vi "pxie_7962_dram_as_memory_fpga.vi"() -> ()   [LabVIEW 2014]
uses:
  <vilib>/Platform/TimedLoop/XDataNode/XDataNode.xnode
  <vilib>/Platform/TimedLoop/XDataNode/nitl_modes.ctl
  <vilib>/Platform/TimedLoop/XDataNode/XDNodeRunTimeDep.lvlib
  <vilib>/Platform/TimedLoop/XDataNode/wakeup.ctl
  <vilib>/Platform/TimedLoop/XDataNode/timing_clust.ctl
  <instrlib>/_niInstr/Streaming/v1/FPGA/niInstr Streaming v1 FPGA.lvlib
  <vilib>/rvi/DataTransferAndStorage/Container/XNode/niFpgaContainer.xnode
  <vilib>/rvi/FIFO/Fifo_Resource/niFpgaFifoEmulationRefIn.vi
  FPGA_Controls/Acquisition FIFOs Cluster.ctl
  <vilib>/eio/EIONode/EIONode.xnode
  <vilib>/rvi/eio/common/nirviEmuTemplateMethod_errors.vi
  <instrlib>/_niInstr/Basic Elements/v1/FPGA/niInstr Basic Elements v1 FPGA.lvlib
  <instrlib>/_niInstr/Streaming/v1/Common/Stream State.ctl
  <instrlib>/_niInstr/Streaming/v1/Common/niInstr Streaming v1 Common.lvlib
  <instrlib>/_niInstr/Basic Elements/v1/FPGA/Private/Count Up U64.vi
  <vilib>/rvi/interface/RandomDataEmulation/nirviRandomDataFpgaReadWriteTemplate.vi
  <vilib>/rvi/FIFO/Fifo_Resource/nirvififoEmulationWrite.vi
panel:
  in  "trigger \ncount":u64
  in  "Clear Trigger":bool
  in  "Debug":bool
  out "stream.metadata 0":u64
  in  "stream.request state 0":T1
  out "stream.samples transferred 0":u64
  out "stream.state 0":T1
  in  "stream.num samples 0":u64
  out "stream 1 \nidle state":bool
  out "stream 1 finite\ntransfer state":bool
  out "stream 1\ncancel state":bool
  out "stream 1\nnot ready state":bool
  out "stream 1\nerror state":bool
  out "Stream 1 data invalid":bool
  out "Writes to DMA":u64
  out "Writes to bundeling FIFO":u64
  out "Samples Aquired":u64
  out "Init Done":bool
  in  "stream.num samples 1":u64
  out "stream.state 1":T1
  out "stream.samples transferred 1":u64
  in  "stream.request state 1":T1
  out "stream.metadata 1":u64
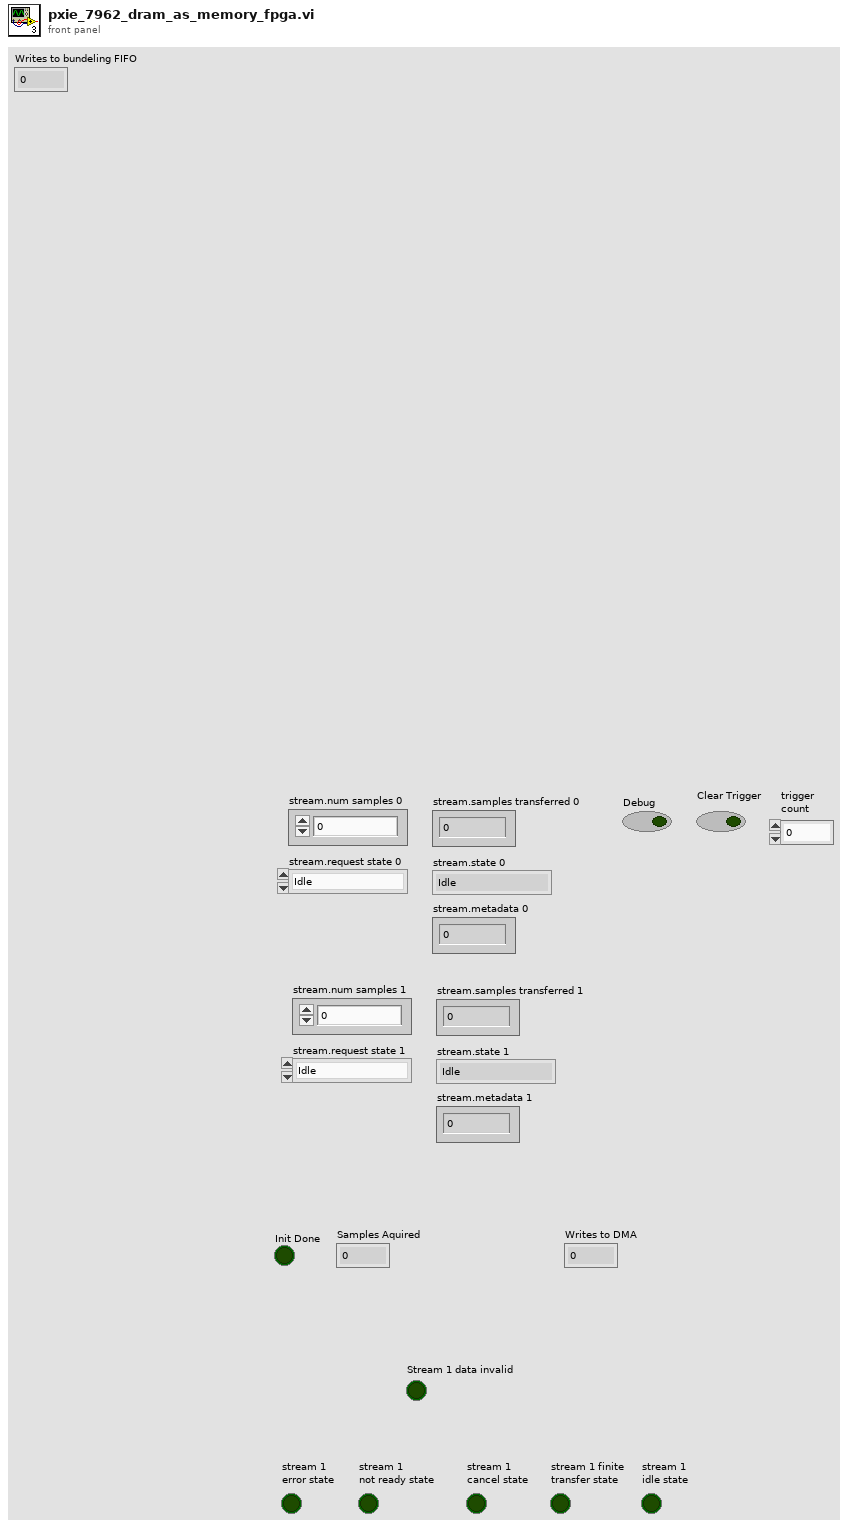
[diagram p1: front panel]
types:
  T1 = typedef "niInstr Streaming v1 Common.lvlib/Stream State.ctl" = enum8{"Idle", "Finite Transfer", "Continuous", "Done", "Error", "Not Ready", "Cancel"}
  T2 = typedef "XDNodeRunTimeDep.lvlib/timing_clust.ctl" = cluster{"Expected End [f-1]":u64, "Actual End [f-1]":u64, "Finished Late? [f-1]":bool, "Expected End [i-1]":u64, "Actual End [i-1]":u64, "Finished Late? [i-1]":bool, "Expected Start [i]":u64, "Actual Start [i]":u64, "Expected Start [f]":u64, "Actual Start [f]":u64, "Source Name":string, "Structure Name":string, "Period":i64, "Deadline":i64, "Offset":i64, "Start":i64, "Priority":i32, "Timeout":i32, "Mode":T3, "Wakeup Reason":T4, "Error":errorcluster, "Source Type":string, "Secondary Source Type":string, "Global End Time":u64, "Global Start Time":u64, "Frame Duration":u64, "Iteration Duration":u64, "Assigned CPU":i32, "I/O Scan Engine Mode":u32}
  T3 = typedef "XDNodeRunTimeDep.lvlib/nitl_modes.ctl" = enum32{"No Change", "Process missed periods, maintain original phase", "Discard missed periods, maintain original phase", "Process missed periods, ignore original phase", "Discard missed periods, ignore original phase"}
  T4 = typedef "XDNodeRunTimeDep.lvlib/wakeup.ctl" = enum32{"Normal", "Aborted", "Asynchronous wakeup", "Timing source error", "Timed loop error", "Timeout"}
  T5 = typedef "Acquisition FIFOs Cluster.ctl" = cluster{"FIFO 0":refnum<k21>, "FIFO 1":refnum<k21>, "FIFO 2":refnum<k21>, "FIFO 3":refnum<k21>, "FIFO 4":refnum<k21>, "FIFO 5":refnum<k21>, "FIFO 6":refnum<k21>, "FIFO 7":refnum<k21>}
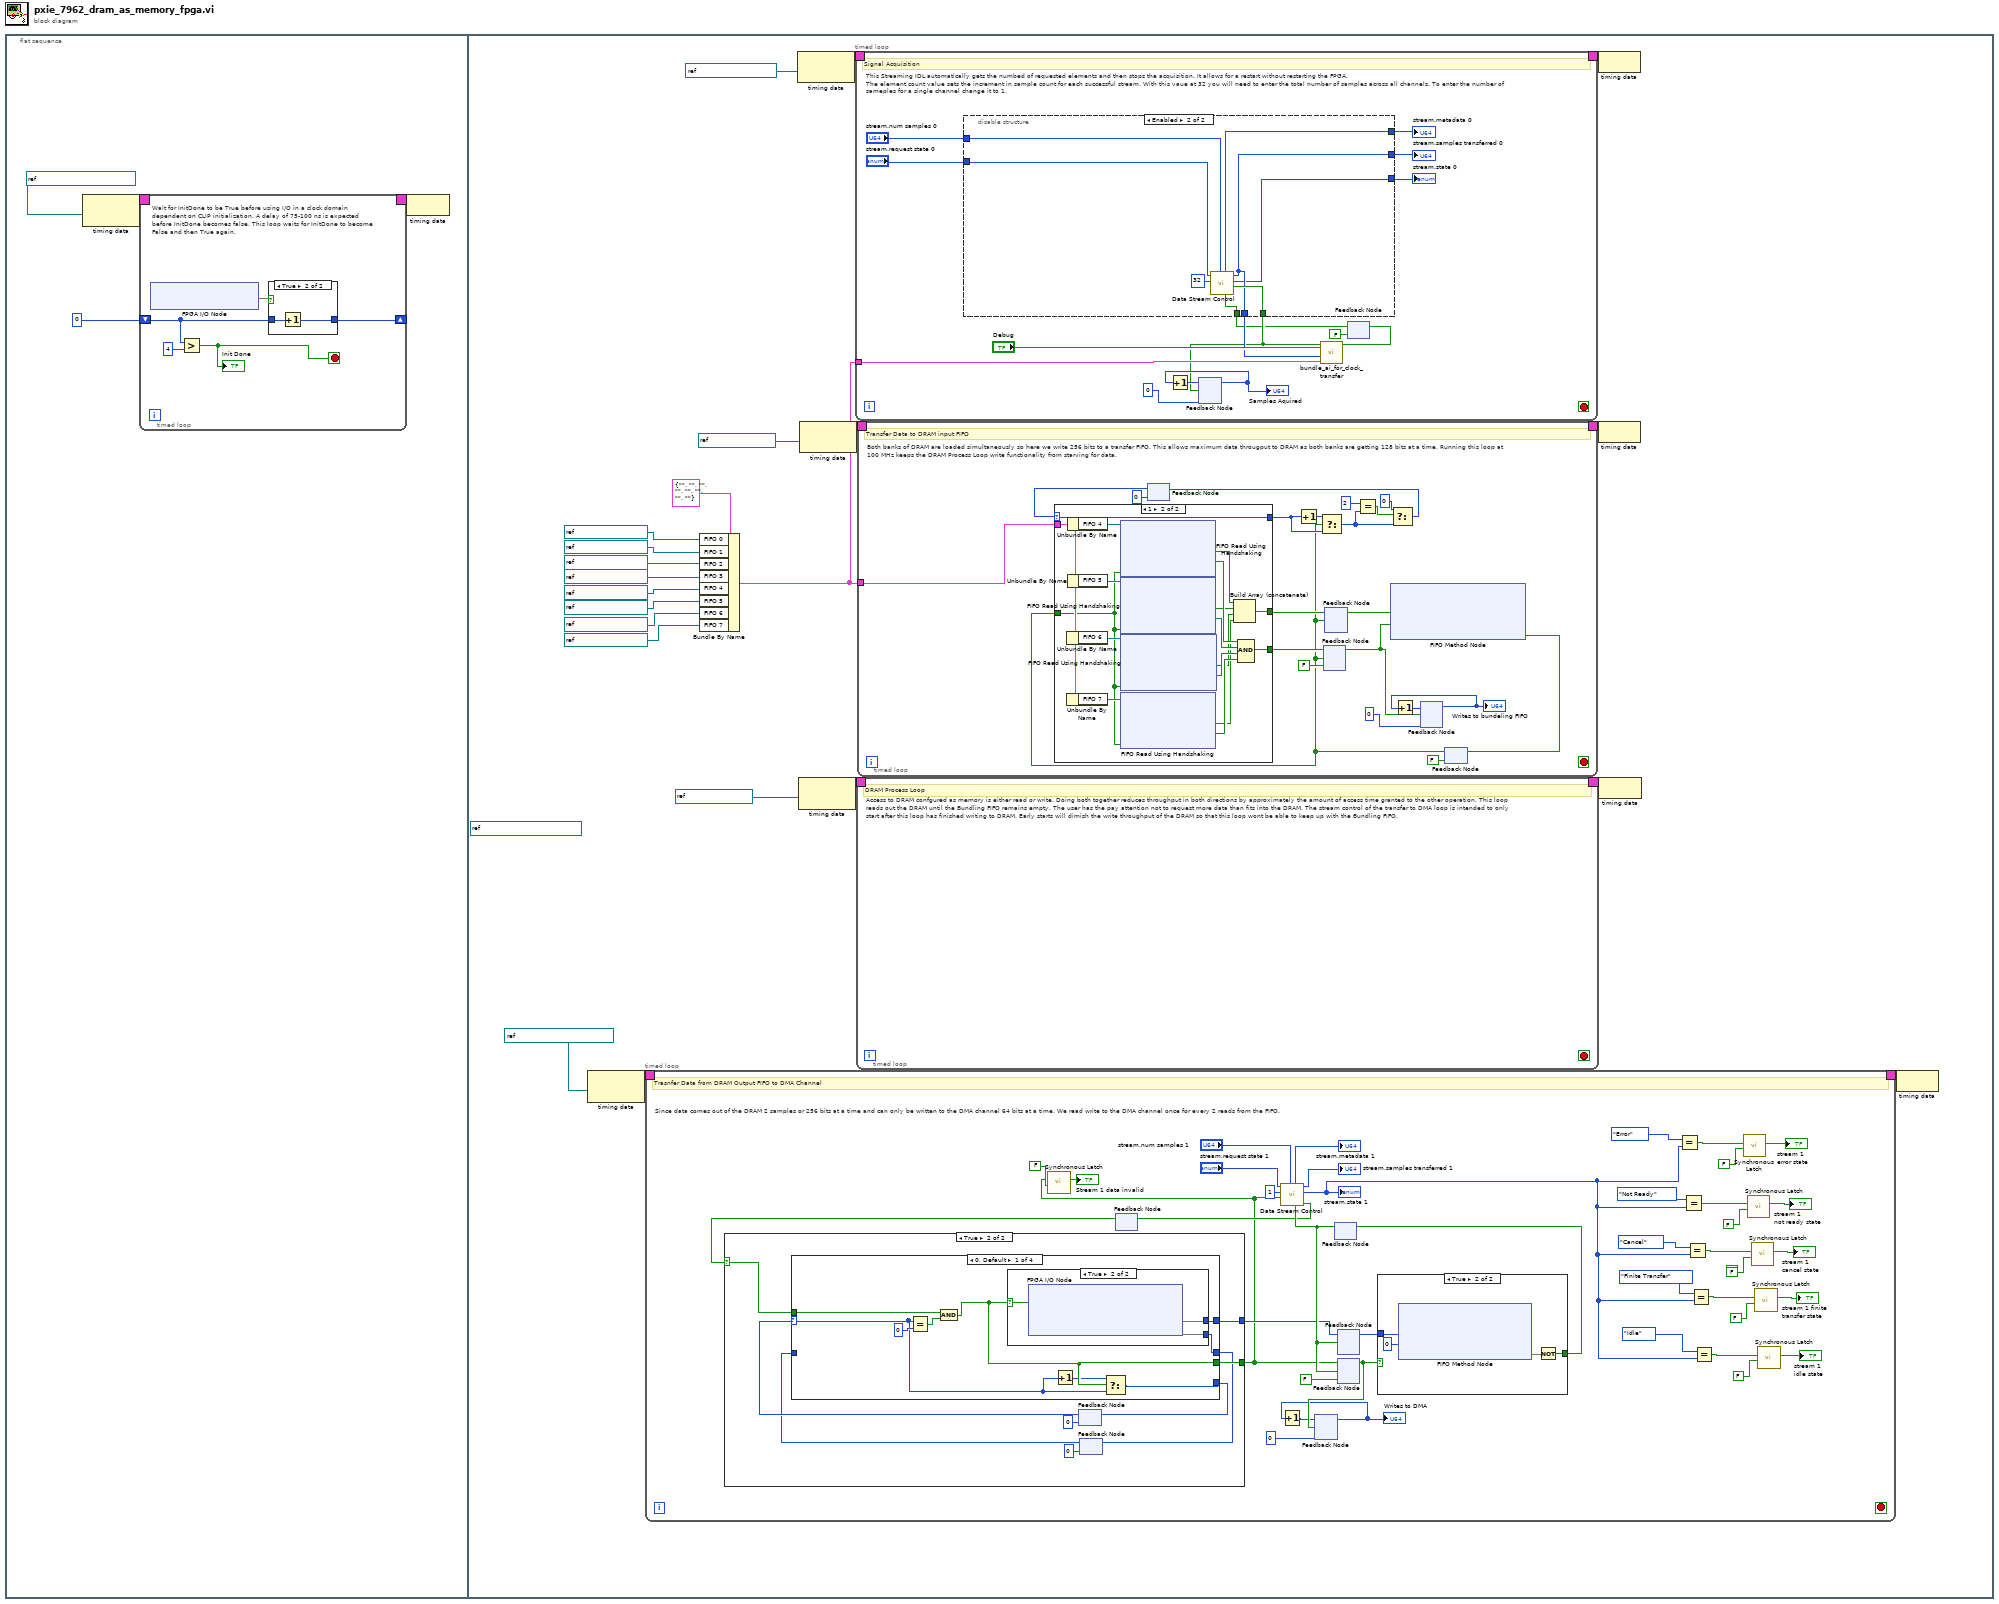
[diagram p0: block diagram]
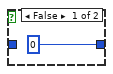
[diagram p2: hidden frame]
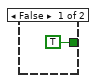
[diagram p3: hidden frame]
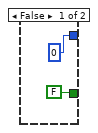
[diagram p4: hidden frame]
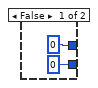
[diagram p5: hidden frame]
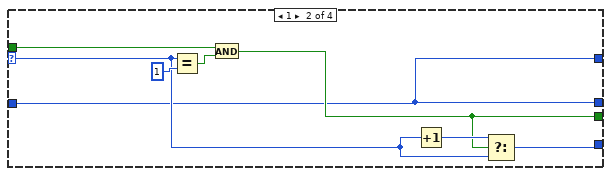
[diagram p6: hidden frame]
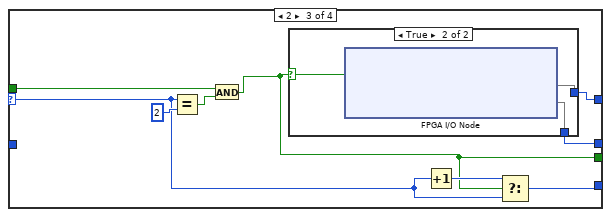
[diagram p7: hidden frame]
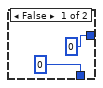
[diagram p8: hidden frame]
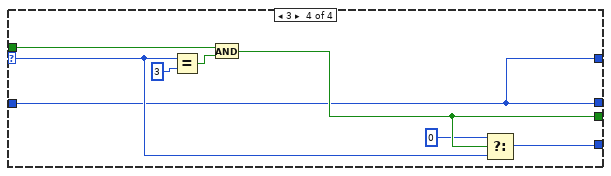
[diagram p9: hidden frame]
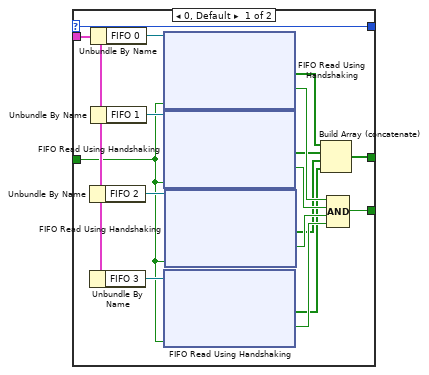
[diagram p10: hidden frame]
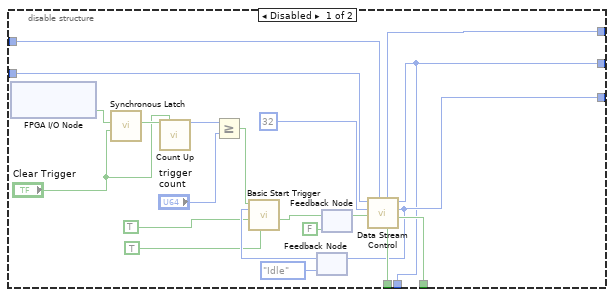
[diagram p11: hidden frame]
diagram:
  n1 = flat-sequence {
    frame #0 {
      n2 = node-c288(refnum<k21> "40 MHz Onboard Clock" ("Source Name")) -> (w4:T2)
      n3 = timed-loop {
        shift-right: [w8] -> _
        shift-left: u16 0 -> [w7]
        timing: w4 -> [_]
        timing-out: [_] -> w3
        stop <- w5 stop-if-true
        # "Wait for InitDone to be True before using I/O in a clock domain dependent on CLIP initialization. A delay of 75-100 ns is expected before InitDone becomes false. This loop waits for InitDone to become False and then True again."
        n4 = xnode "FPGA I/O Node"() -> ("IO Module\\InitDone"=w9)  [unwired: 1 in, 1 out]
        n5 = Greater?(x=w7, y=u16 4) -> (0:w5:bool)
        "Init Done" <- w5
        n6 = case shown="True" w9 {
          tunnel: [u16 0 w12] -> w8
          tunnel: w7 -> [_ w11]
          frame False {
          }
          frame True {
            n7 = Increment(x=w11) -> (x+1=w12:u16)
          }
        }
      }
      n8 = node-c288(w3) -> ()
    }
    frame #1 {
      (unwired) refnum<k21> "Bundling to DRAM FIFO" ("FIFO In")
      n9 = node-c288(refnum<k21> "40 MHz Onboard Clock" ("Source Name")) -> (w34:T2)
      n10 = timed-loop {
        timing: w34 -> [_]
        timing-out: [_] -> w33
        stop <- _ stop-if-true
        (unwired) FALSE ("clear")
        # "Since data comes out of the DRAM 2 samples or 256 bits at a time and can only be written to the DMA channel 64 bits at a time. We read write to the DMA channel once for every 2 reads from the FIFO."
        # "Trasnfer Data from DRAM Output FIFO to DMA Channel"
        n11 = feedback #1() -> (w71:bool)  [unwired: 1 in]
        n12 = case shown="True" w71 {
          selector: w71 -> [_ w92]
          tunnel: [u64 0 ("DRAM Bank 1\\Read_Data_Lower") w96] -> w69
          tunnel: [FALSE w91] -> w62
          frame False {
          }
          frame True {
            n13 = feedback #2(i16 0) -> (w94:i16)
            n14 = feedback #3(u64 0 ("DRAM Bank 1\\Read_Data_Lower")) -> (w89:u64)
            n15 = case shown="0, Default" w94 {
              selector: w94 -> [w98 w113 w120 w135]
              tunnel: w92 -> [w103 w116 w125 w138]
              tunnel: [w102 w111 w124 w133] -> w96
              tunnel: [w101 w112 w122 w134] -> w95
              tunnel: [w100 w114 w121 w137] -> w91
              tunnel: [w97 w111 w119 w133] -> w90
              tunnel: w89 -> [_ w111 _ w133]
              frame 0, Default {
                n16 = Equal?(x=w98, y=i16 0) -> (x = y?=w104:bool)
                n17 = And(x=w103, y=w104) -> (x .and. y?=w100:bool)
                n18 = case shown="True" w100 {
                  selector: w100 -> [_ w109]
                  tunnel: [u64 0 ("DRAM Bank 0\\Read_Data_Upper") w110] -> w102
                  tunnel: [u64 0 ("DRAM Bank 0\\Read_Data_Lower") w108] -> w97
                  frame False {
                  }
                  frame True {
                    n19 = xnode "FPGA I/O Node"("DRAM Bank 0\\Read"=w109) -> ("DRAM Bank 0\\Read_Data_Upper"=w110, "DRAM Bank 0\\Read_Data_Lower"=w108)  [unwired: 3 in, 3 out]
                  }
                }
                n20 = Increment(x=w98) -> (x+1=w99:i16)
                n21 = Select(t=w99, s=w100, f=w98) -> (s? t:f=w101:i16)
              }
              frame 1 {
                n22 = Equal?(x=w113, y=i16 1) -> (x = y?=w117:bool)
                n23 = And(x=w116, y=w117) -> (x .and. y?=w114:bool)
                n24 = Increment(x=w113) -> (x+1=w115:i16)
                n25 = Select(t=w115, s=w114, f=w113) -> (s? t:f=w112:i16)
              }
              frame 2 {
                n26 = Equal?(x=w120, y=i16 2) -> (x = y?=w126:bool)
                n27 = And(x=w125, y=w126) -> (x .and. y?=w121:bool)
                n28 = case shown="True" w121 {
                  selector: w121 -> [_ w132]
                  tunnel: [u64 0 ("DRAM Bank 1\\Read_Data_Upper") w131] -> w124
                  tunnel: [u64 0 ("DRAM Bank 1\\Read_Data_Lower") w130] -> w119
                  frame False {
                  }
                  frame True {
                    n29 = xnode "FPGA I/O Node"("DRAM Bank 1\\Read"=w132) -> ("DRAM Bank 1\\Read_Data_Upper"=w131, "DRAM Bank 1\\Read_Data_Lower"=w130)  [unwired: 3 in, 3 out]
                  }
                }
                n30 = Increment(x=w120) -> (x+1=w123:i16)
                n31 = Select(t=w123, s=w121, f=w120) -> (s? t:f=w122:i16)
              }
              frame 3 {
                n32 = Equal?(x=w135, y=i16 3) -> (x = y?=w139:bool)
                n33 = And(x=w138, y=w139) -> (x .and. y?=w137:bool)
                n34 = Select(t=i16 0, s=w137, f=w135) -> (s? t:f=w134:i16)
              }
            }
            n35 = feedback-in #2(w95) -> ()
            n36 = feedback-in #3(w90) -> ()
          }
        }
        n37 = call <instrlib>:"Synchronous Latch.vi"("clear"=FALSE, "set"=w62) -> ("out"=→"Stream 1 data invalid":bool)  [unwired: 9 in]
        n38 = feedback #4(u64 0) -> (w65:u64)
        "Writes to DMA" <- w65
        n39 = Increment(x=w65) -> (x+1=w66:u64)
        n40 = feedback #5() -> (w73:bool)  [unwired: 1 in]
        n41 = call <instrlib>:"Data Stream Control.vi"("ready for input?"=w73, "stream.num samples 0"="stream.num samples 1", "data valid"=w62, "element count"=u16 1, "stream.request state 0"="stream.request state 1") -> ("request data"=w72:bool, "stream.state 0"=w41:T1, "stream.samples transferred 0"=→"stream.samples transferred 1":u64, "stream.metadata 0"=→"stream.metadata 1":u64)  [unwired: 2 in, 1 out]
        "stream.state 1" <- w41
        n42 = feedback-in #1(w72) -> ()
        n43 = feedback-in #6(w69, w73) -> ()
        n44 = feedback #6() -> (w80:u64)  [unwired: 1 in]
        n45 = feedback #7(FALSE ("Output Valid")) -> (w67:bool)
        n46 = feedback-in #4(w66, w67) -> ()
        n47 = feedback-in #7(w62, w73) -> ()
        n48 = case shown="True" w67 {
          tunnel: w80 -> [_ w85]
          tunnel: [TRUE w83] -> w70
          frame False {
          }
          frame True {
            n49 = xnode ("FIFO Method Node")("Element"=w85, "Timeout"=0) -> ("Timed Out?"=w84)  [unwired: 1 in, 1 out]
            n50 = Not(x=w84) -> (.not. x?=w83:bool)
          }
        }
        n51 = feedback-in #5(w70) -> ()
        n52 = Equal?(x=Stream_State."Error" ("stream.state 0"), y=w41) -> (x = y?=w58:bool)
        n53 = Equal?(x=Stream_State."Not Ready" ("stream.state 0"), y=w41) -> (x = y?=w54:bool)
        n54 = Equal?(x=Stream_State."Cancel" ("stream.state 0"), y=w41) -> (x = y?=w50:bool)
        n55 = Equal?(x=Stream_State."Finite Transfer" ("stream.state 0"), y=w41) -> (x = y?=w46:bool)
        n56 = Equal?(x=Stream_State."Idle" ("stream.state 0"), y=w41) -> (x = y?=w43:bool)
        n57 = call <instrlib>:"Synchronous Latch.vi"("clear"=FALSE, "set"=w58) -> ("out"=→"stream 1\nerror state":bool)  [unwired: 9 in]
        n58 = call <instrlib>:"Synchronous Latch.vi"("clear"=FALSE, "set"=w54) -> ("out"=→"stream 1\nnot ready state":bool)  [unwired: 9 in]
        n59 = call <instrlib>:"Synchronous Latch.vi"("clear"=FALSE, "set"=w50) -> ("out"=→"stream 1\ncancel state":bool)  [unwired: 9 in]
        n60 = call <instrlib>:"Synchronous Latch.vi"("clear"=FALSE, "set"=w46) -> ("out"=→"stream 1 finite\ntransfer state":bool)  [unwired: 9 in]
        n61 = call <instrlib>:"Synchronous Latch.vi"("clear"=FALSE, "set"=w43) -> ("out"=→"stream 1 \nidle state":bool)  [unwired: 9 in]
      }
      n62 = Bundle By Name(cluster=T5 {"FIFO 0"="", "FIFO 1"="", "FIFO 2"="", "FIFO 3"="", "FIFO 4"="", "FIFO 5"="", "FIFO 6"="", "FIFO 7"=""} ("FIFO Refs"), "FIFO 0"=refnum<k21> "AI Bundle FIFO 0" ("FIFO In"), "FIFO 1"=refnum<k21> "AI Bundle FIFO 1" ("FIFO In"), "FIFO 2"=refnum<k21> "AI Bundle FIFO 2" ("FIFO In"), "FIFO 3"=refnum<k21> "AI Bundle FIFO 3" ("FIFO In"), "FIFO 4"=refnum<k21> "AI Bundle FIFO 4" ("FIFO In"), "FIFO 5"=refnum<k21> "AI Bundle FIFO 5" ("FIFO In"), "FIFO 6"=refnum<k21> "AI Bundle FIFO 6" ("FIFO In"), "FIFO 7"=refnum<k21> "AI Bundle FIFO 7" ("FIFO In")) -> (w23:T5)
      n63 = node-c288(refnum<k21> "IO Module Clock 0" ("Source Name")) -> (w40:T2)
      n64 = node-c288(refnum<k21> "100 MHz Clock" ("Source Name")) -> (w36:T2)
      n65 = node-c288(refnum<k21> "100 MHz Clock" ("Source Name")) -> (w38:T2)
      n66 = timed-loop {
        timing: w40 -> [_]
        timing-out: [_] -> w39
        tunnel: w23 -> [w223]
        stop <- _ stop-if-true
        # "This Streaming IDL automatically gets the numbed of requested elements and then stops the acquisition. It allows for a restart without restarting the FPGA. \nThe element count value sets the increment in sample count for each successful stream. With this vaue at 32 you will need to enter the total number of samples across all channels. To enter the number of sameples for a single channel change it to 1."
        # "Signal Acquisition"
        n67 = feedback #8(u64 0) -> (w224:u64)
        "Samples Aquired" <- w224
        n68 = Increment(x=w224) -> (x+1=w225:u64)
        n69 = feedback #9(FALSE ("Ready for Input")) -> (w219:bool)
        n70 = disable-structure shown="Enabled" {
          disable-tunnel: [w238 w253] -> w221
          disable-tunnel: [w248 w256] -> w220
          disable-tunnel: w219 -> [w240 w255]
          disable-tunnel: [w237 w254] -> w218
          disable-tunnel: [w238 w253] -> w217
          disable-tunnel: [w239 w252] -> w216
          disable-tunnel: "stream.num samples 0" -> [w235 w251]
          disable-tunnel: "stream.request state 0" -> [w236 w250]
          frame Disabled {
            n71 = xnode "FPGA I/O Node"() -> ("PXI_Star"=w234:bool)  [unwired: 1 in, 1 out]
            n72 = call <instrlib>:"Synchronous Latch.vi"("clear"="Clear Trigger", "set"=w234) -> ("out"=w233:bool)  [unwired: 9 in]
            n73 = call-poly <instrlib>:"Count Up.vi"("increment"=w233, "reset"="Clear Trigger") -> ("count out"=w232:u64)  [unwired: 13 in]
            n74 = Greater Or Equal?(x=w232, y="trigger \ncount") -> (x >= y?=w231:bool)
            n75 = feedback #10(Stream_State."Idle" ("stream.state 0")) -> (w247:T1)
            n76 = call <instrlib>:"Basic Start Trigger.vi"("ready for start trigger"=TRUE, "data valid?"=TRUE, "stream.state"=w247, "start trigger"=w231) -> ("data valid"=w243:bool)  [unwired: 7 in]
            n77 = feedback #11(FALSE ("data valid")) -> (w244:bool)
            n78 = feedback-in #11(w243) -> ()
            n79 = call <instrlib>:"Data Stream Control.vi"("ready for input?"=w240, "stream.num samples 0"=w235, "data valid"=w244, "element count"=u16 32, "stream.request state 0"=w236) -> ("send data"=w248:bool, "stream.state 0"=w239:T1, "stream.samples transferred 0"=w238:u64, "stream.metadata 0"=w237:u64)  [unwired: 2 in, 1 out]
            n80 = feedback-in #10(w239) -> ()
          }
          frame Enabled {
            n81 = call <instrlib>:"Data Stream Control.vi"("ready for input?"=w255, "stream.num samples 0"=w251, "element count"=u16 32, "stream.request state 0"=w250) -> ("send data"=w256:bool, "stream.state 0"=w252:T1, "stream.samples transferred 0"=w253:u64, "stream.metadata 0"=w254:u64)  [unwired: 3 in, 1 out]
          }
        }
        "stream.state 0" <- w216
        "stream.samples transferred 0" <- w217
        "stream.metadata 0" <- w218
        n82 = feedback-in #8(w225, w220) -> ()
        n83 = call "bundle_ai_for_clock_transfer.vi"("FIFO Refs"=w223, "sample"=w221, "Debug"="Debug", "Input Valid"=w220) -> ("Ready for Input"=w228:bool)  [unwired: 7 in]
        n84 = feedback-in #9(w228) -> ()
      }
      n85 = timed-loop {
        timing: w36 -> [_]
        timing-out: [_] -> w35
        stop <- _ stop-if-true
        # "Access to DRAM confgured as memory is either read or write. Doing both together reduces throughput in both directions by approximately the amount of access time granted to the other operation. This loop reads out the DRAM until the Bundling FIFO remains empty. The user has the pay attention not to request more data than fits into the DRAM. The stream control of the transfer to DMA loop is intended to only start after this loop has finished writing to DRAM. Early starts will dimish the write throughput of the DRAM so that this loop wont be able to keep up with the Bundling FIFO."
        # "DRAM Process Loop"
      }
      n86 = timed-loop {
        timing: w38 -> [_]
        timing-out: [_] -> w37
        tunnel: w23 -> [w173]
        stop <- _ stop-if-true
        # "Both banks of DRAM are loaded simultaneously so here we write 256 bits to a transfer FIFO. This allows maximum data througput to DRAM as both banks are getting 128 bits at a time. Running this loop at 100 MHz keeps the DRAM Process Loop write functionality from starving for data."
        # "Transfer Data to DRAM input FIFO"
        n87 = feedback #12(i16 0 ("t")) -> (w172:i16)
        n88 = feedback #13(FALSE ("Output Valid")) -> (w155:bool)
        n89 = feedback #14() -> (w158:bool[])  [unwired: 1 in]
        n90 = xnode ("FIFO Method Node")("Element"=w158, "Input Valid"=w155) -> ("Ready for Input"=w159:bool)  [unwired: 1 in, 1 out]
        n91 = feedback #15(u64 0) -> (w153:u64)
        "Writes to bundeling FIFO" <- w153
        n92 = Increment(x=w153) -> (x+1=w154:u64)
        n93 = feedback-in #15(w154, w155) -> ()
        n94 = feedback-in #16(w159) -> ()
        n95 = feedback #16(FALSE ("Ready for Input")) -> (w157:bool)
        n96 = case shown="1" w172 {
          selector: w172 -> [w189 w206]
          tunnel: w173 -> [w175 w192]
          tunnel: [w187 w204] -> w160
          tunnel: [w180 w197] -> w171
          tunnel: [w189 w206] -> w167
          tunnel: w157 -> [w174 w191]
          frame 0, Default {
            n97 = Unbundle By Name(w175) -> ("FIFO 2"=w186:refnum<k21>)
            n98 = Unbundle By Name(w175) -> ("FIFO 3"=w185:refnum<k21>)
            n99 = Unbundle By Name(w175) -> ("FIFO 0"=w190:refnum<k21>)
            n100 = Unbundle By Name(w175) -> ("FIFO 1"=w188:refnum<k21>)
            n101 = xnode ("FIFO Read Using Handshaking")("Ready for Output"=w174, "FIFO In"=w190) -> ("Element"=w179:bool[], "Output Valid"=w184:bool)  [unwired: 1 out]
            n102 = xnode ("FIFO Read Using Handshaking")("Ready for Output"=w174, "FIFO In"=w188) -> ("Element"=w178:bool[], "Output Valid"=w183:bool)  [unwired: 1 out]
            n103 = xnode ("FIFO Read Using Handshaking")("Ready for Output"=w174, "FIFO In"=w185) -> ("Element"=w176:bool[], "Output Valid"=w181:bool)  [unwired: 1 out]
            n104 = xnode ("FIFO Read Using Handshaking")("Ready for Output"=w174, "FIFO In"=w186) -> ("Element"=w177:bool[], "Output Valid"=w182:bool)  [unwired: 1 out]
            n105 = Build Array (concatenate)(w179, w178, w177, w176) -> (w187:bool[])
            n106 = Compound Arithmetic op=AND(w184, w183, w182, w181) -> (w180:bool)
          }
          frame 1 {
            n107 = Unbundle By Name(w192) -> ("FIFO 6"=w203:refnum<k21>)
            n108 = Unbundle By Name(w192) -> ("FIFO 7"=w202:refnum<k21>)
            n109 = Unbundle By Name(w192) -> ("FIFO 4"=w207:refnum<k21>)
            n110 = Unbundle By Name(w192) -> ("FIFO 5"=w205:refnum<k21>)
            n111 = xnode ("FIFO Read Using Handshaking")("Ready for Output"=w191, "FIFO In"=w207) -> ("Element"=w196:bool[], "Output Valid"=w201:bool)  [unwired: 1 out]
            n112 = xnode ("FIFO Read Using Handshaking")("Ready for Output"=w191, "FIFO In"=w205) -> ("Element"=w195:bool[], "Output Valid"=w200:bool)  [unwired: 1 out]
            n113 = xnode ("FIFO Read Using Handshaking")("Ready for Output"=w191, "FIFO In"=w202) -> ("Element"=w193:bool[], "Output Valid"=w198:bool)  [unwired: 1 out]
            n114 = xnode ("FIFO Read Using Handshaking")("Ready for Output"=w191, "FIFO In"=w203) -> ("Element"=w194:bool[], "Output Valid"=w199:bool)  [unwired: 1 out]
            n115 = Build Array (concatenate)(w196, w195, w194, w193) -> (w204:bool[])
            n116 = Compound Arithmetic op=AND(w201, w200, w199, w198) -> (w197:bool)
          }
        }
        n117 = Increment(x=w167) -> (x+1=w168:i16)
        n118 = Select(t=w168, s=w157, f=w167) -> (s? t:f=w165:i16)
        n119 = feedback-in #13(w171, w157) -> ()
        n120 = feedback-in #14(w160, w157) -> ()
        n121 = Equal?(x=i16 2, y=w165) -> (x = y?=w164:bool)
        n122 = Select(t=i16 0, s=w164, f=w165) -> (s? t:f=w163:i16)
        n123 = feedback-in #12(w163) -> ()
      }
      n124 = node-c288(w39) -> ()
      n125 = node-c288(w37) -> ()
      n126 = node-c288(w35) -> ()
      n127 = node-c288(w33) -> ()
    }
  }
